vi "Global.vi"() -> ()   [LabVIEW 2017, in "nifxpmath_SinAndCos.xnode"]
uses:
  <vilib>/rvi/FXPMathLib/FxpSinAndCos/XNode/nifxpmath_SinAndCos.xnode
panel:
  in  "TERM Z NAME w/o UNIT":string="x"
  out "SMALL ICON w/ 4WIRE":picture
  in  "TERM C NAME":string="cos(x)"
  in  "TERM S NAME":string="sin(x)"
  in  "TERM Z NAME":string="x (pi)"
  out "SMALL ICON":picture
  in  "TERM C ID":string="TERM_C"
  in  "TERM S ID":string="TERM_S"
  in  "TERM Z ID":string="TERM_Z"
  out "NORMAL BANNER":picture
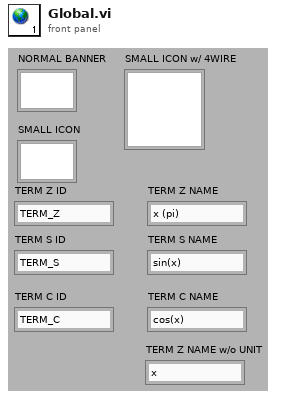
[diagram p1: front panel]
diagram:
